vi "TCP Factory.vi"(8 "error in (no error)":errorcluster, 10 "settings":T1) -> (0 "error out":errorcluster, 3 "protocol out":refnum<class "Protocol Parent.lvclass">)   [LabVIEW 2018, in "Instrument Addon Scripting API.lvlib"]
doc: "Instantiates a new TCP Protocol object using the provided TCP settings."
uses:
  Instrument Addon Scripting API.lvlib
  Addon/Support Libraries/Protocols.lvlibp/TCP/TCP Settings.ctl
  Addon/Support Libraries/Protocols.lvlibp/Protocol Parent/Protocol Parent.lvclass
  Addon/Support Libraries/Protocols.lvlibp/TCP/TCP.lvclass
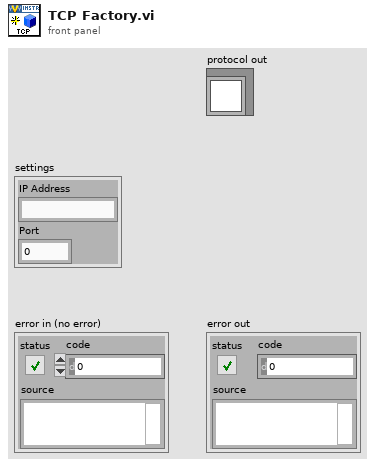
[diagram p1: front panel]
types:
  T1 = typedef "Protocols.lvlibp/TCP.lvclass/TCP Settings.ctl" = cluster{"IP Address":string, "Port":u16}
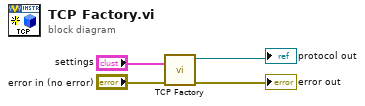
[diagram p0: block diagram]
diagram:
  n1 = call "TCP Factory.vi"("error in (no error)"="error in (no error)", "TCP settings"="settings") -> ("error out"=→"error out":errorcluster, "protocol out"=→"protocol out":refnum<class "Protocol Parent.lvclass">)  [unwired: 8 in]
